vi "Autonomous Independent.vi"() -> ()   [LabVIEW 2018]
doc: "This VI is called when autonomous begins, and will automatically be terminated when autonomous ends. You can carry out timed or sensor driven robot movement independently without needing to return to the caller."
uses:
  <vilib>/Rock Robotics/WPI/Utilities/WPI_GetSetVariantRefNum.vi
  <vilib>/Rock Robotics/Network Tables/NT Read String.vi
  <vilib>/Rock Robotics/Network Tables/NT Write Numeric Array.vi
  <vilib>/Rock Robotics/Network Tables/NT Read Number.vi
  <vilib>/Rock Robotics/Network Tables/NT Write Number.vi
  <vilib>/addons/control/pid/pid.llb/PID (DBL).vi
  <vilib>/Rock Robotics/WPI/ThirdParty/Phoenix-LabVIEW/Pigeon IMU/CTRE_PigeonIMU_GetYPR.vi
  <vilib>/addons/control/pid/NI_PID_pid.lvlib
panel:
  in  "ScaleSpeed":dbl=1.0
  in  "reverse encoder":bool=TRUE
  in  "reverse steer":bool=TRUE
  out "Speed Front Left":dbl
  out "Angle Front Left":dbl
  out "Speed Front Right":dbl
  out "Angle Front Right":dbl
  out "Speed Back Left":dbl
  out "Angle Back Left":dbl
  out "Speed Back Right":dbl
  out "Angle Back Right":dbl
  out "BR Encoder":dbl
  out "BL Encoder":dbl
  out "FL Encoder":dbl
  out "FR  Encoder":dbl
  # "Be sure to right-click and choose Data Operations>>Make Current Value default if you want to save the array values with the VI"
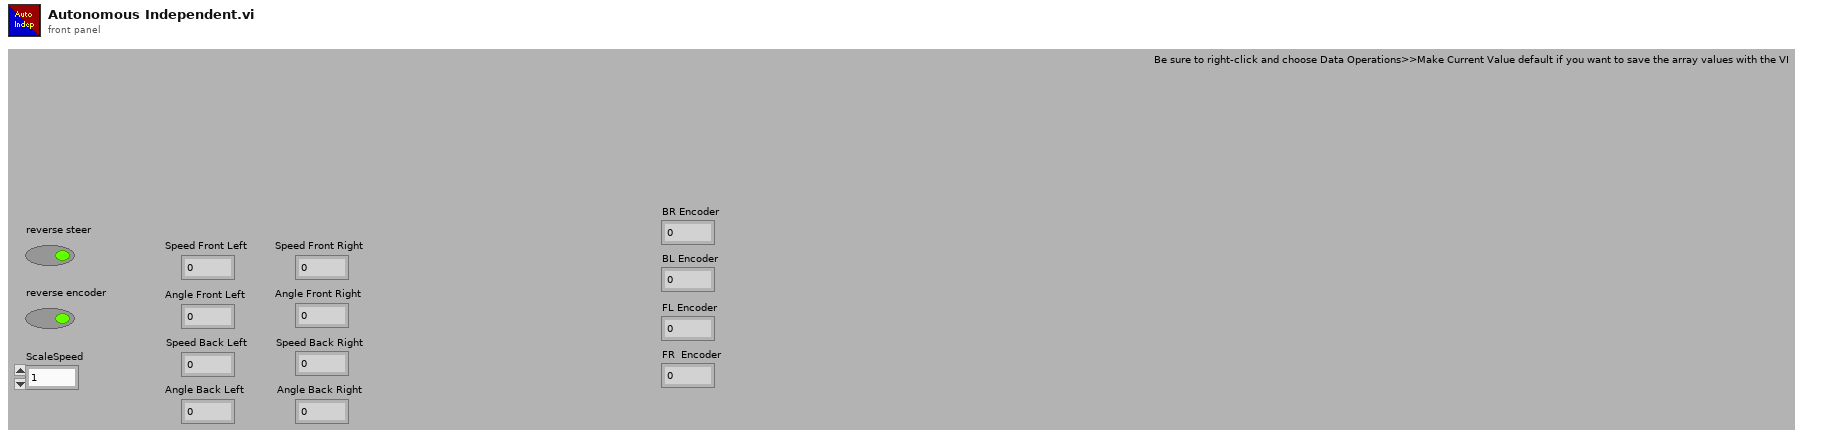
[diagram p1: front panel]
types:
  T1 = typedef "WPI_JoystickDevRef.ctl" = cluster{"Device":T2}
  T2 = typedef "WPI_JoystickDeviceEnum.ctl" = enum16{"USB 0", "USB 1", "USB 2", "USB 3", "USB 4", "USB 5"}
  T3 = cluster{"proportional gain (Kc)":dbl, "integral time (Ti, min)":dbl, "derivative time (Td, min)":dbl}
  T4 = typedef "WPI_MotorControlDeviceRef.ctl" = cluster{"DeviceStatus":errorcluster, "Type":T5, "PWM":cluster{"PWM Channel":T6, "DeadBand":T7}, "CAN":cluster{"Device Number":u8, "SetOutput VI Ref":variant, "GetOutput VI Ref":variant, "Enable VI Ref":variant, "Disable VI Ref":variant, "Data":variant}, "Invert":bool, "DIO PWM":cluster{"PWM \"Enable\" Channel":T6, "DIOChannel":T8, "PWM Rate":dbl}}
  T5 = typedef "WPI_MotorControlType.ctl" = enum16{"PWM", "CAN", "DIO PWM"}
  T6 = typedef "FPGA_DIOPWMChannel.ctl" = enum8{"PWM 0", "PWM 1", "PWM 2", "PWM 3", "PWM 4", "PWM 5", "PWM 6", "PWM 7", "PWM 8", "PWM 9", "PWM MXP 0", "PWM MXP 1", "PWM MXP 2", "PWM MXP 3", "PWM MXP 4", "PWM MXP 5", "PWM MXP 6", "PWM MXP 7", "PWM MXP 8", "PWM MXP 9", "Invalid"}
  T7 = typedef "WPI_PWMDeadband.ctl" = cluster{"Name":string, "maxPositivePwm":i32, "minPositivePwm":i32, "centerPwm":i32, "maxNegativePwm":i32, "minNegativePwm":i32, "angularRange":u16}
  T8 = typedef "FPGA_DIOChannel.ctl" = enum8{"DIO 0", "DIO 1", "DIO 2", "DIO 3", "DIO 4", "DIO 5", "DIO 6", "DIO 7", "DIO 8", "DIO 9", "DIO MXP 0", "DIO MXP 1", "DIO MXP 2", "DIO MXP 3", "DIO MXP 4", "DIO MXP 5", "DIO MXP 6", "DIO MXP 7", "DIO MXP 8", "DIO MXP 9", "DIO MXP 10", "DIO MXP 11", "DIO MXP 12", "DIO MXP 13", "DIO MXP 14", "DIO MXP 15", "SPI Port CS1", "SPI Port CS2", "SPI Port CS3", "SPI Port MISO", "SPI Port MOSI", "Invalid"}
  T9 = typedef "CTRE_PigeonIMU_DeviceRef.ctl" = cluster{"DeviceStatus":errorcluster, "Device Number":u8, "Type":T10, "Device ID":u32, "Handle":u64, "UsageFrame":u32, "Library Path":path}
  T10 = typedef "CTRE_PigeonIMU_ConnectionType.ctl" = u32
  T11 = typedef "WPI_AnalogChannelDevRef.ctl" = cluster{"DevStatus":errorcluster, "Analog Channel":T12}
  T12 = typedef "FPGA_AIChannel.ctl" = enum8{"AI 0", "AI 1", "AI 2", "AI 3", "AI MXP 0", "AI MXP 1", "AI MXP 2", "AI MXP 3", "Invalid"}
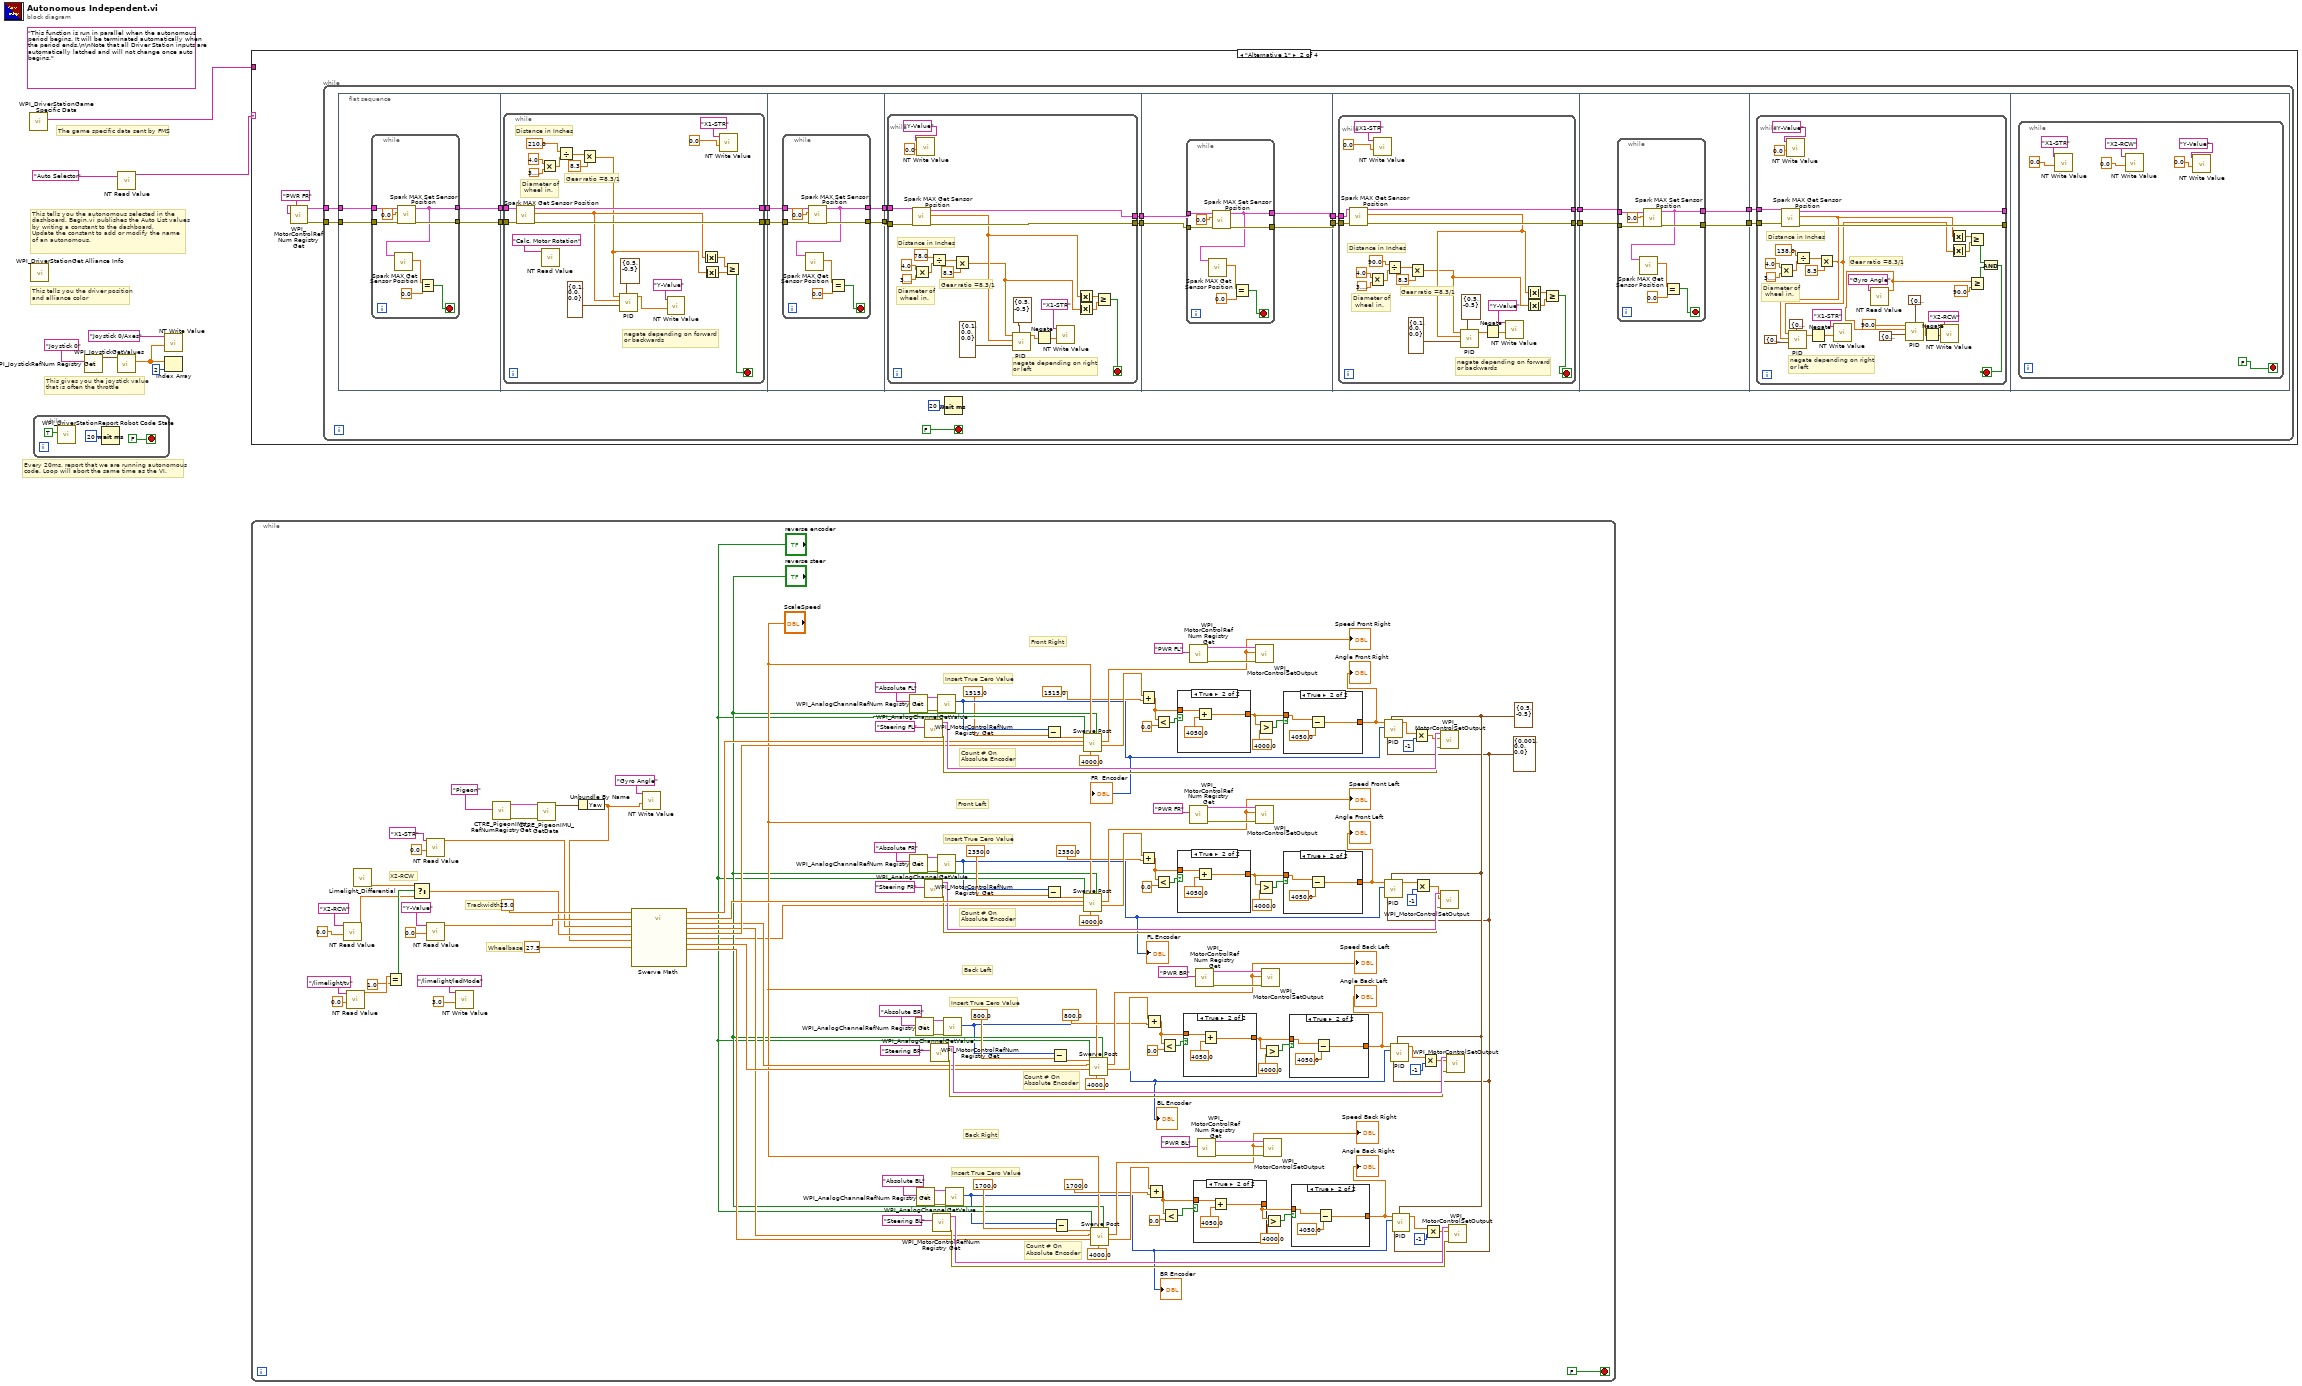
[diagram p0: block diagram]
diagram:
  (unwired) "This function is run in parallel when the autonomous period begins. It will be terminated automatically when the period ends.\n\nNote that all Driver Station inputs are automatically latched and will not change once auto begins."
  # "The game specific data sent by FMS"
  # "This tells you the autonomous selected in the \ndashboard. Begin.vi publishes the Auto List values\nby writing a constant to the dashboard.\nUpdate the constant to add or modify the name\nof an autonomous."
  # "Every 20ms, report that we are running autonomous\ncode. Loop will abort the same time as the VI."
  # "This gives you the joystick value\nthat is often the throttle"
  # "This tells you the driver position\nand alliance color"
  n1 = call <vilib>:"WPI_DriverStationGame Specific Data.vi"() -> ("Game Specific Data"=w1:string)  [unwired: 11 in]
  n2 = call <vilib>:"WPI_DriverStationGet Alliance Info.vi"() -> ()  [unwired: 12 out]
  n3 = while {
    stop <- FALSE stop-if-true
    n4 = call <vilib>:"WPI_DriverStationReport Robot Code State.vi"("Autonomous"=TRUE) -> ()  [unwired: 10 in, 1 out]
    n5 = Wait (ms)(milliseconds to wait=u32 20) -> ()  [unwired: 1 out]
  }
  n6 = call <vilib>:"WPI_JoystickRefNum Registry Get.vi"("refnum name"="Joystick 0") -> ("JoystickDevRef"=w7:T1)  [unwired: 1 in, 9 out]
  n7 = call <vilib>:"WPI_JoystickGetValues.vi"("JoystickDevRef"=w7) -> ("Axes"=w4:dbl[])  [unwired: 6 in, 4 out]
  n8 = call-poly <vilib>:"NT Read Value.vi"("Name"="Auto Selector") -> ("String"=w2:string)  [unwired: 9 in, 1 out]
  n9 = call-poly <vilib>:"NT Write Value.vi"("Numeric Array"=w4, "Name"="Joystick 0/Axes") -> ()  [unwired: 9 in, 1 out]
  n10 = Index Array(array=w4, index=2) -> ()  [unwired: 1 out]
  n11 = case shown="\"Alternative 1\"" w2 {
    tunnel: w1 -> [_ _ _ _]
    frame Default {
    }
    frame "Alternative 1" {
      n12 = call <vilib>:"WPI_MotorControlRefNum Registry Get.vi"("refnum name"="PWR FR") -> ("error out"=w13:errorcluster, "MotorControlDevRef"=w14:T4)  [unwired: 9 in]
      n13 = while {
        tunnel: w13 -> [w30]
        tunnel: w14 -> [w31]
        stop <- FALSE stop-if-true
        n14 = flat-sequence {
          tunnel: w30 -> [w35]
          tunnel: w31 -> [w36]
          tunnel: [w34] -> w24
          tunnel: [w33] -> w23
          tunnel: [w46] -> w28
          tunnel: [w45] -> w27
          tunnel: w24 -> [w48]
          tunnel: w23 -> [w47]
          tunnel: w28 -> [w72]
          tunnel: w27 -> [w74]
          tunnel: [w73] -> w26
          tunnel: [w71] -> w25
          tunnel: w26 -> [w86]
          tunnel: [w85] -> w22
          tunnel: [w84] -> w20
          tunnel: w25 -> [w83]
          tunnel: w22 -> [w110]
          tunnel: [w112] -> w21
          tunnel: w20 -> [w109]
          tunnel: [w111] -> w19
          tunnel: w21 -> [w124]
          tunnel: w19 -> [w123]
          tunnel: [w122] -> w18
          tunnel: [w121] -> w16
          tunnel: w18 -> [w148]
          tunnel: [w150] -> w17
          tunnel: w16 -> [w147]
          tunnel: [w149] -> w15
          tunnel: w17 -> [w160]
          tunnel: w15 -> [w159]
          frame #0 {
            n15 = while {
              tunnel: w36 -> [w44]
              tunnel: [w40] -> w34
              tunnel: w35 -> [w43]
              tunnel: [w42] -> w33
              stop <- w37 stop-if-true
              n16 = call <vilib>:"Spark MAX Set Sensor Position.vi"("error in"=w43, "Position"=0.0, "MotorControlDeviceRef"=w44) -> ("error out"=w42:errorcluster, "MotorControlDeviceRef"=w40:T4)  [unwired: 7 in]
              n17 = call <vilib>:"Spark MAX Get Sensor Position.vi"("MotorControlDevRef in"=w40) -> ("Sensor Position"=w38:dbl)  [unwired: 7 in, 3 out]
              n18 = Equal?(x=w38, y=0.0) -> (x = y?=w37:bool)
            }
          }
          frame #1 {
            n19 = while {
              tunnel: w47 -> [w70]
              tunnel: w48 -> [w69]
              tunnel: [w68] -> w45
              tunnel: [w67] -> w46
              stop <- w63 stop-if-true
              # "Distance in Inches"
              # "Diameter of\n wheel in."
              # "Gear ratio =8.3/1"
              # "negate depending on forward \nor backwards"
              n20 = call <vilib>:"Spark MAX Get Sensor Position.vi"("error in (no error)"=w70, "MotorControlDevRef in"=w69) -> ("error out"=w67:errorcluster, "Sensor Position"=w59:dbl, "MotorControlDevRef out"=w68:T4)  [unwired: 6 in, 1 out]
              n21 = Multiply(x=4.0, y=3.141592653589793) -> (x*y=w55:dbl)
              n22 = call-poly <vilib>:"NT Read Value.vi"("Name"="Calc. Motor Rotation") -> ()  [unwired: 9 in, 2 out]
              n23 = Divide(x=210.0, y=w55) -> (x/y=w54:dbl)
              n24 = Multiply(x=w54, y=8.3) -> (x*y=w49:dbl)
              n25 = call-poly <vilib>:"PID.vi"("output range"=cluster{"output high":dbl, "output low":dbl} {"output high"=0.5, "output low"=-0.5} ("output range 2"), "PID gains"=T3 {"proportional gain (Kc)"=0.1, "integral time (Ti, min)"=0.0, "derivative time (Td, min)"=0.0} ("PID gains 2"), "process variable"=w59, "setpoint"=w49) -> ("output"=w56:dbl)  [unwired: 6 in, 1 out]
              n26 = call-poly <vilib>:"NT Write Value.vi"("Numeric"=w56, "Name"="Y-Value") -> ()  [unwired: 9 in, 1 out]
              n27 = Absolute Value(x=w59) -> (abs(x)=w60:dbl)
              n28 = Absolute Value(x=w49) -> (abs(x)=w61:dbl)
              n29 = call-poly <vilib>:"NT Write Value.vi"("Numeric"=0.0, "Name"="X1-STR") -> ()  [unwired: 9 in, 1 out]
              n30 = Greater Or Equal?(x=w60, y=w61) -> (x >= y?=w63:bool)
            }
          }
          frame #2 {
            n31 = while {
              tunnel: w74 -> [w82]
              tunnel: [w78] -> w73
              tunnel: w72 -> [w81]
              tunnel: [w80] -> w71
              stop <- w75 stop-if-true
              n32 = call <vilib>:"Spark MAX Set Sensor Position.vi"("error in"=w81, "Position"=0.0, "MotorControlDeviceRef"=w82) -> ("error out"=w80:errorcluster, "MotorControlDeviceRef"=w78:T4)  [unwired: 7 in]
              n33 = call <vilib>:"Spark MAX Get Sensor Position.vi"("MotorControlDevRef in"=w78) -> ("Sensor Position"=w76:dbl)  [unwired: 7 in, 3 out]
              n34 = Equal?(x=w76, y=0.0) -> (x = y?=w75:bool)
            }
          }
          frame #3 {
            n35 = while {
              tunnel: w86 -> [w108]
              tunnel: [w103] -> w85
              tunnel: [w102] -> w84
              tunnel: w83 -> [w95]
              stop <- w104 stop-if-true
              # "Gear ratio =8.3/1"
              # "Diameter of\n wheel in."
              # "Distance in Inches"
              # "negate depending on right \nor left"
              n36 = call <vilib>:"Spark MAX Get Sensor Position.vi"("error in (no error)"=w95, "MotorControlDevRef in"=w108) -> ("error out"=w102:errorcluster, "Sensor Position"=w96:dbl, "MotorControlDevRef out"=w103:T4)  [unwired: 6 in, 1 out]
              n37 = Multiply(x=4.0, y=3.141592653589793) -> (x*y=w93:dbl)
              n38 = call-poly <vilib>:"NT Write Value.vi"("Numeric"=0.0, "Name"="Y-Value") -> ()  [unwired: 9 in, 1 out]
              n39 = Divide(x=78.0, y=w93) -> (x/y=w92:dbl)
              n40 = Multiply(x=w92, y=8.3) -> (x*y=w87:dbl)
              n41 = call-poly <vilib>:"PID.vi"("output range"=cluster{"output high":dbl, "output low":dbl} {"output high"=0.5, "output low"=-0.5} ("output range 2"), "PID gains"=T3 {"proportional gain (Kc)"=0.1, "integral time (Ti, min)"=0.0, "derivative time (Td, min)"=0.0} ("PID gains 2"), "process variable"=w96, "setpoint"=w87) -> ("output"=w99:dbl)  [unwired: 6 in, 1 out]
              n42 = Negate(x=w99) -> (-x=w94:dbl)
              n43 = call-poly <vilib>:"NT Write Value.vi"("Numeric"=w94, "Name"="X1-STR") -> ()  [unwired: 9 in, 1 out]
              n44 = Absolute Value(x=w96) -> (abs(x)=w98:dbl)
              n45 = Absolute Value(x=w87) -> (abs(x)=w97:dbl)
              n46 = Greater Or Equal?(x=w98, y=w97) -> (x >= y?=w104:bool)
            }
          }
          frame #4 {
            n47 = while {
              tunnel: w110 -> [w120]
              tunnel: [w116] -> w112
              tunnel: w109 -> [w119]
              tunnel: [w118] -> w111
              stop <- w113 stop-if-true
              n48 = call <vilib>:"Spark MAX Set Sensor Position.vi"("error in"=w119, "Position"=0.0, "MotorControlDeviceRef"=w120) -> ("error out"=w118:errorcluster, "MotorControlDeviceRef"=w116:T4)  [unwired: 7 in]
              n49 = call <vilib>:"Spark MAX Get Sensor Position.vi"("MotorControlDevRef in"=w116) -> ("Sensor Position"=w114:dbl)  [unwired: 7 in, 3 out]
              n50 = Equal?(x=w114, y=0.0) -> (x = y?=w113:bool)
            }
          }
          frame #5 {
            n51 = while {
              tunnel: w124 -> [w143]
              tunnel: w123 -> [w142]
              tunnel: [w141] -> w122
              tunnel: [w140] -> w121
              stop <- w133 stop-if-true
              # "Distance in Inches"
              # "Gear ratio =8.3/1"
              # "Diameter of\n wheel in."
              # "negate depending on forward \nor backwards"
              n52 = call <vilib>:"Spark MAX Get Sensor Position.vi"("error in (no error)"=w142, "MotorControlDevRef in"=w143) -> ("error out"=w140:errorcluster, "Sensor Position"=w135:dbl, "MotorControlDevRef out"=w141:T4)  [unwired: 6 in, 1 out]
              n53 = Multiply(x=4.0, y=3.141592653589793) -> (x*y=w131:dbl)
              n54 = call-poly <vilib>:"NT Write Value.vi"("Numeric"=0.0, "Name"="X1-STR") -> ()  [unwired: 9 in, 1 out]
              n55 = Divide(x=90.0, y=w131) -> (x/y=w130:dbl)
              n56 = Multiply(x=w130, y=8.3) -> (x*y=w126:dbl)
              n57 = call-poly <vilib>:"PID.vi"("output range"=cluster{"output high":dbl, "output low":dbl} {"output high"=0.5, "output low"=-0.5} ("output range 2"), "PID gains"=T3 {"proportional gain (Kc)"=0.1, "integral time (Ti, min)"=0.0, "derivative time (Td, min)"=0.0} ("PID gains 2"), "process variable"=w135, "setpoint"=w126) -> ("output"=w134:dbl)  [unwired: 6 in, 1 out]
              n58 = Negate(x=w134) -> (-x=w132:dbl)
              n59 = call-poly <vilib>:"NT Write Value.vi"("Numeric"=w132, "Name"="Y-Value") -> ()  [unwired: 9 in, 1 out]
              n60 = Absolute Value(x=w135) -> (abs(x)=w137:dbl)
              n61 = Absolute Value(x=w126) -> (abs(x)=w136:dbl)
              n62 = Greater Or Equal?(x=w137, y=w136) -> (x >= y?=w133:bool)
            }
          }
          frame #6 {
            n63 = while {
              tunnel: w148 -> [w158]
              tunnel: [w154] -> w150
              tunnel: w147 -> [w157]
              tunnel: [w156] -> w149
              stop <- w151 stop-if-true
              n64 = call <vilib>:"Spark MAX Set Sensor Position.vi"("error in"=w157, "Position"=0.0, "MotorControlDeviceRef"=w158) -> ("error out"=w156:errorcluster, "MotorControlDeviceRef"=w154:T4)  [unwired: 7 in]
              n65 = call <vilib>:"Spark MAX Get Sensor Position.vi"("MotorControlDevRef in"=w154) -> ("Sensor Position"=w152:dbl)  [unwired: 7 in, 3 out]
              n66 = Equal?(x=w152, y=0.0) -> (x = y?=w151:bool)
            }
          }
          frame #7 {
            n67 = while {
              tunnel: w160 -> [w193]
              tunnel: w159 -> [w192]
              tunnel: [w188] -> _
              tunnel: [w187] -> _
              stop <- w170 stop-if-true
              # "Gear ratio =8.3/1"
              # "Diameter of\n wheel in."
              # "Distance in Inches"
              # "negate depending on right \nor left"
              n68 = Multiply(x=4.0, y=3.141592653589793) -> (x*y=w167:dbl)
              n69 = call <vilib>:"Spark MAX Get Sensor Position.vi"("error in (no error)"=w192, "MotorControlDevRef in"=w193) -> ("error out"=w187:errorcluster, "Sensor Position"=w181:dbl, "MotorControlDevRef out"=w188:T4)  [unwired: 6 in, 1 out]
              n70 = call-poly <vilib>:"NT Write Value.vi"("Numeric"=0.0, "Name"="Y-Value") -> ()  [unwired: 9 in, 1 out]
              n71 = Divide(x=138.0, y=w167) -> (x/y=w166:dbl)
              n72 = Multiply(x=w166, y=8.3) -> (x*y=w161:dbl)
              n73 = call-poly <vilib>:"PID.vi"("output range"=cluster{"output high":dbl, "output low":dbl} {"output high"=0.5, "output low"=-0.5} ("output range 2"), "PID gains"=T3 {"proportional gain (Kc)"=0.1, "integral time (Ti, min)"=0.0, "derivative time (Td, min)"=0.0} ("PID gains 2"), "process variable"=w181, "setpoint"=w161) -> ("output"=w184:dbl)  [unwired: 6 in, 1 out]
              n74 = Negate(x=w184) -> (-x=w168:dbl)
              n75 = call-poly <vilib>:"NT Write Value.vi"("Numeric"=w168, "Name"="X1-STR") -> ()  [unwired: 9 in, 1 out]
              n76 = call-poly <vilib>:"NT Read Value.vi"("Name"="Gyro Angle") -> ("Numeric"=w169:dbl)  [unwired: 9 in, 1 out]
              n77 = call-poly <vilib>:"PID.vi"("output range"=cluster{"output high":dbl, "output low":dbl} {"output high"=0.5, "output low"=-0.5} ("output range 2"), "PID gains"=T3 {"proportional gain (Kc)"=0.009, "integral time (Ti, min)"=0.0, "derivative time (Td, min)"=0.0} ("PID gains 2"), "process variable"=w169, "setpoint"=90.0) -> ("output"=w171:dbl)  [unwired: 6 in, 1 out]
              n78 = Negate(x=w171) -> (-x=w172:dbl)
              n79 = call-poly <vilib>:"NT Write Value.vi"("Numeric"=w172, "Name"="X2-RCW") -> ()  [unwired: 9 in, 1 out]
              n80 = Absolute Value(x=w181) -> (abs(x)=w183:dbl)
              n81 = Absolute Value(x=w161) -> (abs(x)=w182:dbl)
              n82 = Greater Or Equal?(x=w183, y=w182) -> (x >= y?=w175:bool)
              n83 = Greater Or Equal?(x=w169, y=90.0) -> (x >= y?=w174:bool)
              n84 = And(x=w175, y=w174) -> (x .and. y?=w170:bool)
            }
          }
          frame #8 {
            n85 = while {
              stop <- FALSE stop-if-true
              n86 = call-poly <vilib>:"NT Write Value.vi"("Numeric"=0.0, "Name"="X1-STR") -> ()  [unwired: 9 in, 1 out]
              n87 = call-poly <vilib>:"NT Write Value.vi"("Numeric"=0.0, "Name"="X2-RCW") -> ()  [unwired: 9 in, 1 out]
              n88 = call-poly <vilib>:"NT Write Value.vi"("Numeric"=0.0, "Name"="Y-Value") -> ()  [unwired: 9 in, 1 out]
            }
          }
        }
        n89 = Wait (ms)(milliseconds to wait=u32 20) -> ()  [unwired: 1 out]
      }
    }
    frame "Alternative 2" {
    }
    frame "Your Turn" {
    }
  }
  n90 = while {
    stop <- FALSE stop-if-true
    w248 = cluster{"output high":dbl, "output low":dbl} {"output high"=0.5, "output low"=-0.5} ("output range 2")
    w247 = T3 {"proportional gain (Kc)"=0.001, "integral time (Ti, min)"=0.0, "derivative time (Td, min)"=0.0} ("PID gains 2")
    # "X2-RCW"
    # "Trackwidth"
    # "Wheelbase"
    # "Count # On \nAbsolute Encoder"
    # "Insert True Zero Value"
    # "Count # On \nAbsolute Encoder"
    # "Insert True Zero Value"
    # "Count # On \nAbsolute Encoder"
    # "Insert True Zero Value"
    # "Count # On \nAbsolute Encoder"
    # "Insert True Zero Value"
    # "Back Right"
    # "Back Left"
    # "Front Left"
    # "Front Right"
    n91 = call-poly <vilib>:"NT Read Value.vi"("Default Value"=0.0, "Name"="X2-RCW") -> ("Numeric"=w207:dbl)  [unwired: 8 in, 1 out]
    n92 = call-poly <vilib>:"NT Read Value.vi"("Default Value"=0.0, "Name"="/limelight/tv") -> ("Numeric"=w212:dbl)  [unwired: 8 in, 1 out]
    n93 = call "Limelight_Differential.vi"() -> ("SteerCommand"=w227:dbl)  [unwired: 8 in, 2 out]
    n94 = Equal?(x=w212, y=1.0) -> (x = y?=w210:bool)
    n95 = Select(t=w227, s=w210, f=w207) -> (s? t:f=w213:dbl)
    n96 = call-poly <vilib>:"NT Read Value.vi"("Default Value"=0.0, "Name"="X1-STR") -> ("Numeric"=w216:dbl)  [unwired: 8 in, 1 out]
    n97 = call-poly <vilib>:"NT Read Value.vi"("Default Value"=0.0, "Name"="Y-Value") -> ("Numeric"=w219:dbl)  [unwired: 8 in, 1 out]
    n98 = call-poly <vilib>:"NT Write Value.vi"("Numeric"=3.0, "Name"="/limelight/ledMode") -> ()  [unwired: 9 in, 1 out]
    n99 = call <vilib>:"CTRE_PigeonIMU_RefNumRegistryGet.vi"("refnum name"="Pigeon") -> ("error out"=w225:errorcluster, "PigeonIMUDevRef"=w224:T9)  [unwired: 9 in]
    n100 = call-poly <vilib>:"CTRE_PigeonIMU_GetData.vi"("error in (no error)"=w225, "PigeonIMUDevRef"=w224) -> ("Yaw Pitch Roll"=w223:cluster{"Yaw":dbl, "Pitch":dbl, "Roll":dbl})  [unwired: 7 in, 2 out]
    n101 = Unbundle By Name(w223) -> ("Yaw"=w202:dbl)
    n102 = call "Swerve Math.vi"("Trackwidth (W)"=25.0, "Wheelbase (L)"=27.5, "Y -FWD"=w219, "X1 STR"=w216, "X2 RCW"=w213, "Gyro Angle in degrees"=w202) -> ("wa3"=w280:dbl, "wa4"=w255:dbl, "ws1"=w302:dbl, "ws2"=w342:dbl, "ws3"=w279:dbl, "ws4"=w256:dbl, "wa2"=w230:dbl, "wa1"=w303:dbl)  [unwired: 2 in]
    n103 = call-poly <vilib>:"NT Write Value.vi"("Numeric"=w202, "Name"="Gyro Angle") -> ()  [unwired: 9 in, 1 out]
    n104 = call <vilib>:"WPI_AnalogChannelRefNum Registry Get.vi"("refnum name"="Absolute FL") -> ("error out"=w317:errorcluster, "AIDeviceRef"=w316:T11)  [unwired: 9 in]
    n105 = call <vilib>:"WPI_AnalogChannelRefNum Registry Get.vi"("refnum name"="Absolute FR") -> ("error out"=w338:errorcluster, "AIDeviceRef"=w337:T11)  [unwired: 9 in]
    n106 = call <vilib>:"WPI_AnalogChannelRefNum Registry Get.vi"("refnum name"="Absolute BR") -> ("error out"=w296:errorcluster, "AIDeviceRef"=w295:T11)  [unwired: 9 in]
    n107 = call <vilib>:"WPI_AnalogChannelRefNum Registry Get.vi"("refnum name"="Absolute BL") -> ("error out"=w273:errorcluster, "AIDeviceRef"=w272:T11)  [unwired: 9 in]
    n108 = call <vilib>:"WPI_MotorControlRefNum Registry Get.vi"("refnum name"="Steering FL") -> ("error out"=w311:errorcluster, "MotorControlDevRef"=w312:T4)  [unwired: 9 in]
    n109 = call <vilib>:"WPI_MotorControlRefNum Registry Get.vi"("refnum name"="Steering FR") -> ("error out"=w330:errorcluster, "MotorControlDevRef"=w331:T4)  [unwired: 9 in]
    n110 = call <vilib>:"WPI_MotorControlRefNum Registry Get.vi"("refnum name"="Steering BR") -> ("error out"=w288:errorcluster, "MotorControlDevRef"=w289:T4)  [unwired: 9 in]
    n111 = call <vilib>:"WPI_MotorControlRefNum Registry Get.vi"("refnum name"="Steering BL") -> ("error out"=w265:errorcluster, "MotorControlDevRef"=w266:T4)  [unwired: 9 in]
    n112 = call <vilib>:"WPI_AnalogChannelGetValue.vi"("error in (no error)"=w317, "AIDeviceRef"=w316) -> ("Value"=w249:i16)  [unwired: 7 in, 2 out]
    "FR  Encoder" <- w249
    n113 = call <vilib>:"WPI_AnalogChannelGetValue.vi"("error in (no error)"=w338, "AIDeviceRef"=w337) -> ("Value"=w250:i16)  [unwired: 7 in, 2 out]
    "FL Encoder" <- w250
    n114 = call <vilib>:"WPI_AnalogChannelGetValue.vi"("error in (no error)"=w296, "AIDeviceRef"=w295) -> ("Value"=w251:i16)  [unwired: 7 in, 2 out]
    "BL Encoder" <- w251
    n115 = call <vilib>:"WPI_AnalogChannelGetValue.vi"("error in (no error)"=w273, "AIDeviceRef"=w272) -> ("Value"=w252:i16)  [unwired: 7 in, 2 out]
    "BR Encoder" <- w252
    n116 = Subtract(x=w249, y=1515.0) -> (x-y=w314:dbl)
    n117 = Subtract(x=w250, y=2350.0) -> (x-y=w334:dbl)
    n118 = Subtract(x=w251, y=800.0) -> (x-y=w292:dbl)
    n119 = Subtract(x=w252, y=1700.0) -> (x-y=w269:dbl)
    n120 = call "Swerve Post.vi"("reverse encoder"="reverse encoder", "reverse steer"="reverse steer", "gear ratio"=4000.0, "ScaleSpeed"="ScaleSpeed", "wa in"=w303, "ws in"=w302, "encoder in"=w314) -> ("wa out"=w313:dbl, "ws out 0-1"=w318:dbl)  [unwired: 3 in]
    "Speed Front Right" <- w318
    n121 = call "Swerve Post.vi"("reverse encoder"="reverse encoder", "reverse steer"="reverse steer", "gear ratio"=4000.0, "ScaleSpeed"="ScaleSpeed", "wa in"=w230, "ws in"=w342, "encoder in"=w334) -> ("wa out"=w333:dbl, "ws out 0-1"=w339:dbl)  [unwired: 3 in]
    "Speed Front Left" <- w339
    n122 = call "Swerve Post.vi"("reverse encoder"="reverse encoder", "reverse steer"="reverse steer", "gear ratio"=4000.0, "ScaleSpeed"="ScaleSpeed", "wa in"=w280, "ws in"=w279, "encoder in"=w292) -> ("wa out"=w291:dbl, "ws out 0-1"=w297:dbl)  [unwired: 3 in]
    "Speed Back Left" <- w297
    n123 = call "Swerve Post.vi"("reverse encoder"="reverse encoder", "reverse steer"="reverse steer", "gear ratio"=4000.0, "ScaleSpeed"="ScaleSpeed", "wa in"=w255, "ws in"=w256, "encoder in"=w269) -> ("wa out"=w268:dbl, "ws out 0-1"=w274:dbl)  [unwired: 3 in]
    "Speed Back Right" <- w274
    n124 = Add(x=w313, y=1515.0) -> (x+y=w308:dbl)
    n125 = Add(x=w333, y=2350.0) -> (x+y=w327:dbl)
    n126 = Add(x=w291, y=800.0) -> (x+y=w285:dbl)
    n127 = Add(x=w268, y=1700.0) -> (x+y=w262:dbl)
    n128 = Less?(x=w308, y=0.0) -> (x < y?=w310:bool)
    n129 = Less?(x=w327, y=0.0) -> (x < y?=w329:bool)
    n130 = Less?(x=w285, y=0.0) -> (x < y?=w287:bool)
    n131 = Less?(x=w262, y=0.0) -> (x < y?=w264:bool)
    n132 = case shown="True" w310 {
      tunnel: w308 -> [w365 w368]
      tunnel: [w365 w366] -> w305
      frame False {
      }
      frame True {
        n133 = Add(x=w368, y=4050.0) -> (x+y=w366:dbl)
      }
    }
    n134 = case shown="True" w329 {
      tunnel: w327 -> [w373 w376]
      tunnel: [w373 w374] -> w324
      frame False {
      }
      frame True {
        n135 = Add(x=w376, y=4050.0) -> (x+y=w374:dbl)
      }
    }
    n136 = case shown="True" w287 {
      tunnel: w285 -> [w357 w360]
      tunnel: [w357 w358] -> w282
      frame False {
      }
      frame True {
        n137 = Add(x=w360, y=4050.0) -> (x+y=w358:dbl)
      }
    }
    n138 = call <vilib>:"WPI_MotorControlRefNum Registry Get.vi"("refnum name"="PWR FL") -> ("error out"=w319:errorcluster, "MotorControlDevRef"=w320:T4)  [unwired: 9 in]
    n139 = call <vilib>:"WPI_MotorControlRefNum Registry Get.vi"("refnum name"="PWR FR") -> ("error out"=w340:errorcluster, "MotorControlDevRef"=w341:T4)  [unwired: 9 in]
    n140 = case shown="True" w264 {
      tunnel: w262 -> [w349 w352]
      tunnel: [w349 w350] -> w259
      frame False {
      }
      frame True {
        n141 = Add(x=w352, y=4050.0) -> (x+y=w350:dbl)
      }
    }
    n142 = call <vilib>:"WPI_MotorControlRefNum Registry Get.vi"("refnum name"="PWR BR") -> ("error out"=w298:errorcluster, "MotorControlDevRef"=w299:T4)  [unwired: 9 in]
    n143 = call <vilib>:"WPI_MotorControlRefNum Registry Get.vi"("refnum name"="PWR BL") -> ("error out"=w275:errorcluster, "MotorControlDevRef"=w276:T4)  [unwired: 9 in]
    n144 = call <vilib>:"WPI_MotorControlSetOutput.vi"("error in (no error)"=w319, "Output"=w318, "MotorControlDevRef"=w320) -> ()  [unwired: 6 in, 3 out]
    n145 = call <vilib>:"WPI_MotorControlSetOutput.vi"("error in (no error)"=w340, "Output"=w339, "MotorControlDevRef"=w341) -> ()  [unwired: 6 in, 3 out]
    n146 = Greater?(x=w305, y=4000.0) -> (0:w307:bool)
    n147 = Greater?(x=w324, y=4000.0) -> (0:w326:bool)
    n148 = call <vilib>:"WPI_MotorControlSetOutput.vi"("error in (no error)"=w298, "Output"=w297, "MotorControlDevRef"=w299) -> ()  [unwired: 6 in, 3 out]
    n149 = Greater?(x=w282, y=4000.0) -> (0:w284:bool)
    n150 = call <vilib>:"WPI_MotorControlSetOutput.vi"("error in (no error)"=w275, "Output"=w274, "MotorControlDevRef"=w276) -> ()  [unwired: 6 in, 3 out]
    n151 = Greater?(x=w259, y=4000.0) -> (0:w261:bool)
    n152 = case shown="True" w307 {
      tunnel: w305 -> [w361 w364]
      tunnel: [w361 w362] -> w243
      frame False {
      }
      frame True {
        n153 = Subtract(x=w364, y=4050.0) -> (x-y=w362:dbl)
      }
    }
    "Angle Front Right" <- w243
    n154 = case shown="True" w326 {
      tunnel: w324 -> [w369 w372]
      tunnel: [w369 w370] -> w244
      frame False {
      }
      frame True {
        n155 = Subtract(x=w372, y=4050.0) -> (x-y=w370:dbl)
      }
    }
    "Angle Front Left" <- w244
    n156 = case shown="True" w284 {
      tunnel: w282 -> [w353 w356]
      tunnel: [w353 w354] -> w245
      frame False {
      }
      frame True {
        n157 = Subtract(x=w356, y=4050.0) -> (x-y=w354:dbl)
      }
    }
    "Angle Back Left" <- w245
    n158 = case shown="True" w261 {
      tunnel: w259 -> [w345 w348]
      tunnel: [w345 w346] -> w246
      frame False {
      }
      frame True {
        n159 = Subtract(x=w348, y=4050.0) -> (x-y=w346:dbl)
      }
    }
    "Angle Back Right" <- w246
    n160 = call-poly <vilib>:"PID.vi"("output range"=w248, "PID gains"=w247, "process variable"=w249, "setpoint"=w243) -> ("output"=w232:dbl)  [unwired: 6 in, 1 out]
    n161 = call-poly <vilib>:"PID.vi"("output range"=w248, "PID gains"=w247, "process variable"=w250, "setpoint"=w244) -> ("output"=w242:dbl)  [unwired: 6 in, 1 out]
    n162 = call-poly <vilib>:"PID.vi"("output range"=w248, "PID gains"=w247, "process variable"=w251, "setpoint"=w245) -> ("output"=w235:dbl)  [unwired: 6 in, 1 out]
    n163 = call-poly <vilib>:"PID.vi"("output range"=w248, "PID gains"=w247, "process variable"=w252, "setpoint"=w246) -> ("output"=w238:dbl)  [unwired: 6 in, 1 out]
    n164 = Multiply(x=w232, y=-1) -> (x*y=w233:dbl)
    n165 = Multiply(x=w242, y=-1) -> (x*y=w241:dbl)
    n166 = Multiply(x=w235, y=-1) -> (x*y=w236:dbl)
    n167 = Multiply(x=w238, y=-1) -> (x*y=w239:dbl)
    n168 = call <vilib>:"WPI_MotorControlSetOutput.vi"("error in (no error)"=w311, "Output"=w233, "MotorControlDevRef"=w312) -> ()  [unwired: 6 in, 3 out]
    n169 = call <vilib>:"WPI_MotorControlSetOutput.vi"("error in (no error)"=w330, "Output"=w241, "MotorControlDevRef"=w331) -> ()  [unwired: 6 in, 3 out]
    n170 = call <vilib>:"WPI_MotorControlSetOutput.vi"("error in (no error)"=w288, "Output"=w236, "MotorControlDevRef"=w289) -> ()  [unwired: 6 in, 3 out]
    n171 = call <vilib>:"WPI_MotorControlSetOutput.vi"("error in (no error)"=w265, "Output"=w239, "MotorControlDevRef"=w266) -> ()  [unwired: 6 in, 3 out]
  }
